vi "Build Log Handshake.vi"(7 "Command":string, 8 "error in (no error)":errorcluster, 11 "BuildLog":path) -> (0 "error out":errorcluster)   [LabVIEW 2010]
uses:
  <userlib>/_OpenG.lib/file/file.llb/File Exists - Scalar__ogtk.vi
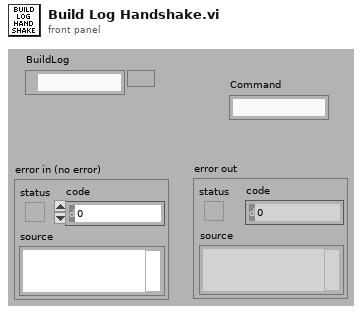
[diagram p1: front panel]
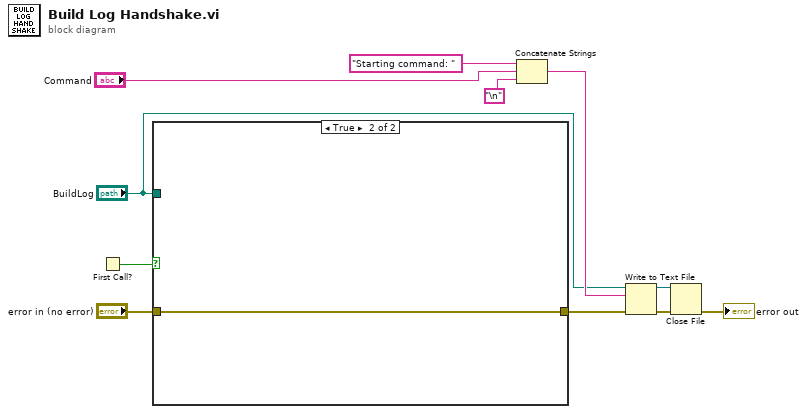
[diagram p0: block diagram]
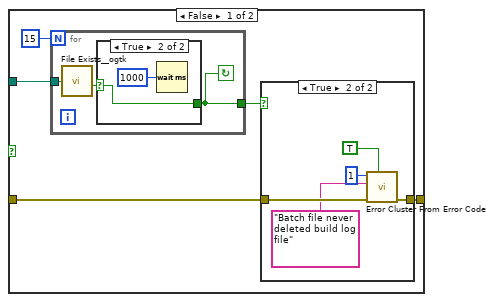
[diagram p2: hidden frame]
diagram:
  n1 = First Call?() -> (First Call?: T/F=w2:bool)
  n2 = case shown="True" w2 {
    tunnel: "error in (no error)" -> [w14 w29]
    tunnel: [w13 w29] -> w10
    tunnel: "BuildLog" -> [w12 _]
    frame False {
      n3 = for {
        N: 15 -> [_]
        tunnel: w12 -> [w25]
        tunnel: [w23] -> w15
        stop <- w23 continue-if-true
        n4 = call-poly <userlib>:"File Exists__ogtk.vi"("file path"=w25) -> ("exists"=w24:bool)  [unwired: 6 in, 1 out]
        n5 = case shown="True" w24 {
          selector: w24 -> [w26 w27]
          tunnel: [w26 w27] -> w23
          frame False {
          }
          frame True {
            n6 = Wait (ms)(milliseconds to wait=u32 1000) -> ()  [unwired: 1 out]
          }
        }
      }
      n7 = case shown="True" w15 {
        tunnel: w14 -> [w17 w22]
        tunnel: [w17 w18] -> w13
        frame False {
        }
        frame True {
          n8 = call <vilib>:"Error Cluster From Error Code.vi"("show call chain? (False)"=TRUE, "error in (no error)"=w22, "error message (\"\")"="Batch file never deleted build log file" ("error message (\"\")"), "error code (0)"=1) -> ("error out"=w18:errorcluster)  [unwired: 5 in]
        }
      }
    }
    frame True {
    }
  }
  n9 = Concatenate Strings("Starting command: " ("string"), "Command", "\n") -> (w7:string)
  n10 = Write to Text File(file (use dialog)="BuildLog", text=w7, error in=w10) -> (refnum out=w4:refnum<file>, error out=w5:errorcluster)  [unwired: 1 in, 1 out]
  n11 = Close File(refnum=w4, error in=w5) -> (error out=→"error out":errorcluster)  [unwired: 1 out]
